vi "Communication - Data Pulse PRun (FGV).vi"(7 "Action":T1=enum."Write", 8 "error in (no error)":errorcluster, 10 "Pulse In":i64[](array[numeric]), 11 "P Run In":bool[](array[boolean])) -> (0 "error out":errorcluster, 2 "Pulse Out":i64[](array[numeric]), 3 "P Run Out":bool[](array[boolean]))   [LabVIEW 2019]
uses:
  Controls/FGV States.ctl
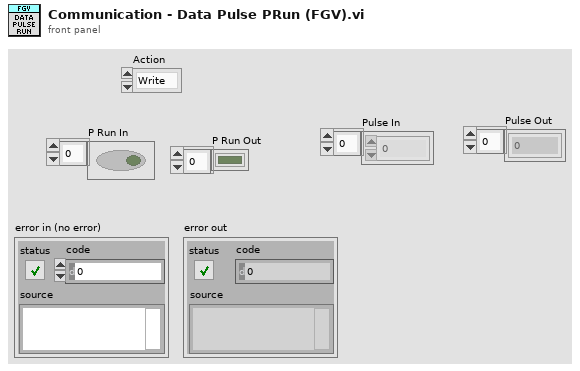
[diagram p1: front panel]
types:
  T1 = typedef "FGV States.ctl" = enum16{"Read", "Write"}
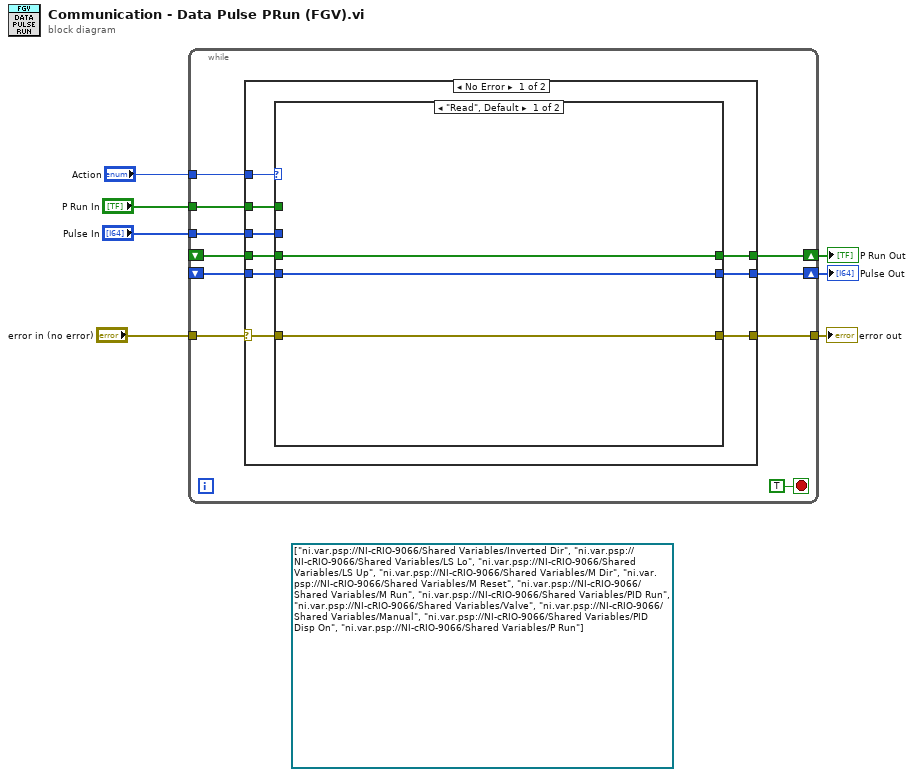
[diagram p0: block diagram]
diagram:
  (unwired) refnum<k21>[] ["ni.var.psp://NI-cRIO-9066/Shared Variables/Inverted Dir", "ni.var.psp://NI-cRIO-9066/Shared Variables/LS Lo", "ni.var.psp://NI-cRIO-9066/Shared Variables/LS Up", "ni.var.psp://NI-cRIO-9066/Shared Variables/M Dir", "ni.var.psp://NI-cRIO-9066/Shared Variables/M Reset", "ni.var.psp://NI-cRIO-9066/Shared Variables/M Run", "ni.var.psp://NI-cRIO-9066/Shared Variables/PID Run", "ni.var.psp://NI-cRIO-9066/Shared Variables/Valve", "ni.var.psp://NI-cRIO-9066/Shared Variables/Manual", "ni.var.psp://NI-cRIO-9066/Shared Variables/PID Disp On", "ni.var.psp://NI-cRIO-9066/Shared Variables/P Run"]
  n1 = while {
    tunnel: "Action" -> [w17]
    tunnel: "P Run In" -> [w15]
    shift-right: [w16] -> w5
    shift-left: _ -> [w14]
    tunnel: "error in (no error)" -> [w12]
    tunnel: [w11] -> w3
    tunnel: "Pulse In" -> [w9]
    shift-right: [w10] -> w1
    shift-left: _ -> [w8]
    stop <- TRUE stop-if-true
    n2 = case shown="No Error" w12 {
      selector: w12 -> [w21 w34]
      tunnel: w17 -> [w26 _]
      tunnel: [w25 w35] -> w16
      tunnel: w15 -> [w24 _]
      tunnel: w14 -> [w23 w35]
      tunnel: [w22 w34] -> w11
      tunnel: [w20 w33] -> w10
      tunnel: w9 -> [w19 _]
      tunnel: w8 -> [w18 w33]
      frame No Error {
        n3 = case shown="\"Read\", Default" w26 {
          tunnel: [w29 w32] -> w25
          tunnel: w24 -> [_ w32]
          tunnel: w23 -> [w29 _]
          tunnel: [w28 w31] -> w22
          tunnel: w21 -> [w28 w31]
          tunnel: [w27 w30] -> w20
          tunnel: w19 -> [_ w30]
          tunnel: w18 -> [w27 _]
          frame "Read", Default {
          }
          frame "Write" {
          }
        }
      }
      frame Error {
      }
    }
  }
  "P Run Out" <- w5
  "error out" <- w3
  "Pulse Out" <- w1
